vi "Tracepoint_StartBurstMode.vi"(8 "error in (no error)":errorcluster, 10 "ForceBurst":bool, 11 "Qbus":refnum<class "Qbus.lvclass">) -> (0 "error out":errorcluster)   [LabVIEW 2017, in "BurstMode.lvlib"]
uses:
  <vilib>/addons/InsightCM/Devices/Shared/Cms/CmsBurstMode/BurstMode.lvlib
  <vilib>/addons/Qbus/Qbus.lvclass
  <vilib>/addons/TraceLogger/TraceLogger.lvlib
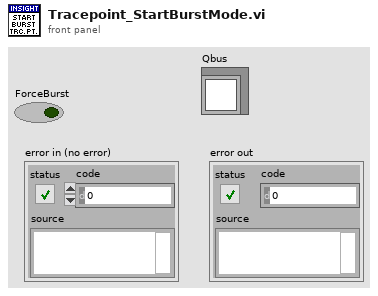
[diagram p1: front panel]
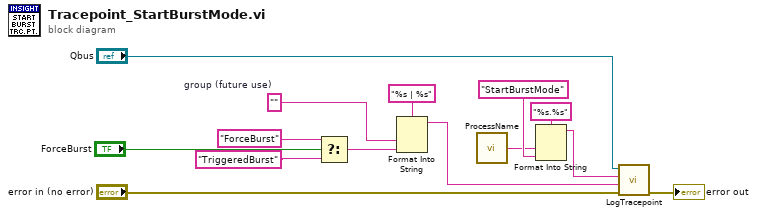
[diagram p0: block diagram]
diagram:
  w1 = ""  # group (future use)
  n1 = Select(t="ForceBurst" ("StreamId"), s="ForceBurst", f="TriggeredBurst" ("StreamId")) -> (s? t:f=w2:string)
  n2 = Format Into String(format string="%s | %s", w1, w2) -> (resulting string=w8:string)  [unwired: 2 in, 1 out]
  n3 = call <vilib>:"ProcessName.vi"() -> ("process name"=w5:string)  [unwired: 5 in]
  n4 = Format Into String(format string="%s.%s", w5, "StartBurstMode" ("tracepoint")) -> (resulting string=w10:string)  [unwired: 2 in, 1 out]
  n5 = call <vilib>:"LogTracepoint.vi"("error in (no error)"="error in (no error)", "log string"=w8, "tracepoint"=w10, "qbus in"="Qbus") -> ("error out"=→"error out":errorcluster)  [unwired: 6 in, 1 out]
